vi "Generate Links.vi"(9 "error in (no error)":errorcluster, 10 "Create Unowned Container?":bool, 11 "Name-Dep array":T1[](array[typedef])) -> (1 "error out":errorcluster, 3 "String":string)   [LabVIEW 2018, in "Name and Dependency Processing.lvlib"]
uses:
  Name and Dependency Processing.lvlib
  Name - Dep Cluster.ctl
  DGML Creation/DGML creation.lvlib
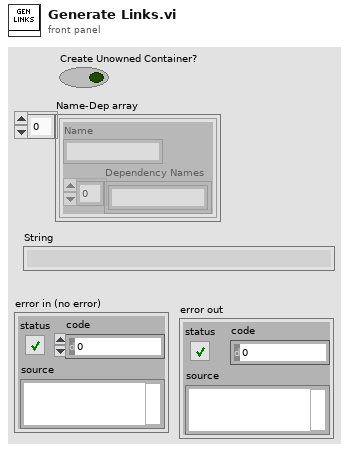
[diagram p1: front panel]
types:
  T1 = typedef "Name and Dependency Processing.lvlib/Name - Dep Cluster.ctl" = cluster{"Name":string, "Dependency Names":string[]}
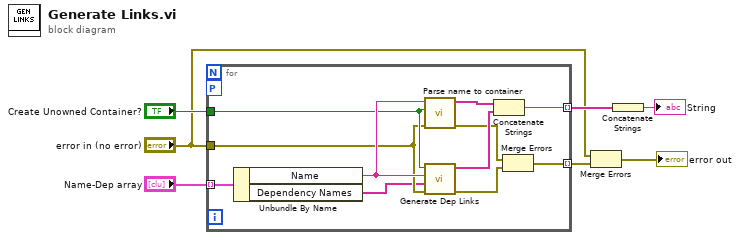
[diagram p0: block diagram]
diagram:
  n1 = for {
    tunnel: "Name-Dep array" -> [w18] mode=indexing
    tunnel: "error in (no error)" -> [w12]
    tunnel: [w17] -> w5 mode=indexing
    workers-P: _ -> [_]
    tunnel: "Create Unowned Container?" -> [w13]
    tunnel: [w9] -> w3 mode=indexing
    n2 = Unbundle By Name(w18) -> ("Name"=w15:string, "Dependency Names"=w8:string[])
    n3 = call "Parse name to container.vi"("error in"=w12, "Create Unowned Container?"=w13, "Fully Qualified Name"=w15) -> ("error out"=w11:errorcluster, "Container DGML Strings"=w14:string[])  [unwired: 7 in]
    n4 = call "Generate Dep Links.vi"("error in"=w12, "Dependency Names"=w8, "Name"=w15, "Create Unowned Container?"=w13) -> ("error out"=w10:errorcluster, "DGML Link Strings"=w16:string[])  [unwired: 6 in]
    n5 = Concatenate Strings(w14, w16) -> (w17:string)
    n6 = Merge Errors(w11, w10) -> (w9:errorcluster)
  }
  n7 = Merge Errors("error in (no error)", w3) -> (→"error out":errorcluster)
  n8 = Concatenate Strings(w5) -> (→"String":string)
